vi "SIAM_test_Standalone.vi"() -> ()   [LabVIEW 2011]
uses:
  SIAM_command.ctl
  Library/ScanControl/ScanControl_Action.ctl
  Library/ScanControl/ScanControl_Channel.ctl
  SIAM-send.ctl
  <vilib>/Utility/miscctls.llb/LVRangeTypeDef.ctl
panel:
  in  "Clear":bool
  in  "return":string="78,0,\r\n78,0,\r\n78,0,\r\n78,0,\r\n78,0,\r\n78,0,\r\n78,0,\r\n78,0,\r\n78,0,\r\n78,0,\r\n78,0,\r\n78,0,\r\n78,0,\r\n78,0,\r\n78,0,\r\n78,0,\r\n78,0,\r\n78,0,\r\n78,0,\r\n78,0,\r\n78,0,\r\n78,0,\r\n78,0,\r\n78,0,\r\n78,0,\r\n78,0,\r\n78,0,\r\n78,0,\r\n"
  in  "Registerkarte":T1(tab)
  in  "ScaleConst":T2(array[cluster])=[{"Axis-Ring"=16777217, "Scale"=51200.0, "Offset"=100.0, "HW min"=0.0, "HW max"=5500000.0, "max a"=inf, "units"="mm"}, {"Axis-Ring"=17825793, "Scale"=51200.0, "Offset"=100.0, "HW min"=0.0, "HW max"=3700000.0, "max a"=inf, "units"="mm"}, {"Axis-Ring"=19922945, "Scale"=153600.0, "Offset"=146600.0, "HW min"=0.0, "HW max"=614400.0, "max a"=inf, "units"="Pos"}, {"Axis-Ring"=20971521, "Scale"=25000.1, "Offset"=641.0, "HW min"=0.0, "HW max"=124721.0, "max a"=inf, "units"="Pos"}, {"Axis-Ring"=22020097, "Scale"=1.0, "Offset"=0.0, "HW min"=0.0, "HW max"=51200.0, "max a"=inf, "units"="counts"}, {"Axis-Ring"=23068673, "Scale"=10240.0, "Offset"=0.0, "HW min"=0.0, "HW max"=51200.0, "max a"=inf, "units"="Pos"}, {"Axis-Ring"=24117249, "Scale"=1.0, "Offset"=0.0, "HW min"=0.0, "HW max"=51200.0, "max a"=inf, "units"="counts"}, {"Axis-Ring"=2684354561, "Scale"=1.0, "Offset"=0.0, "HW min"=0.0, "HW max"=65636.0, "max a"=inf, "units"="counts"}, {"Axis-Ring"=2685403137, "Scale"=1.0, "Offset"=0.0, "HW min"=0.0, "HW max"=65636.0, "max a"=inf, "units"="counts"}, {"Axis-Ring"=2686451713, "Scale"=1.0, "Offset"=0.0, "HW min"=0.0, "HW max"=65636.0, "max a"=inf, "units"="counts"}, {"Axis-Ring"=2687500289, "Scale"=1.0, "Offset"=0.0, "HW min"=0.0, "HW max"=65636.0, "max a"=inf, "units"="counts"}, {"Axis-Ring"=2688548865, "Scale"=1.0, "Offset"=0.0, "HW min"=0.0, "HW max"=65636.0, "max a"=inf, "units"="counts"}, {"Axis-Ring"=2689597441, "Scale"=1.0, "Offset"=1.0, "HW min"=0.0, "HW max"=65636.0, "max a"=inf, "units"="counts"}, {"Axis-Ring"=2690646017, "Scale"=1.0, "Offset"=1.0, "HW min"=0.0, "HW max"=65636.0, "max a"=inf, "units"="counts"}, {"Axis-Ring"=2691694593, "Scale"=1.0, "Offset"=1.0, "HW min"=0.0, "HW max"=65636.0, "max a"=inf, "units"="counts"}, {"Axis-Ring"=2701131777, "Scale"=1.0, "Offset"=1.0, "HW min"=0.0, "HW max"=65636.0, "max a"=inf, "units"="counts"}, {"Axis-Ring"=2702180353, "Scale"=1.0, "Offset"=1.0, "HW min"=0.0, "HW max"=65636.0, "max a"=inf, "units"="counts"}, {"Axis-Ring"=2703228929, "Scale"=1.0, "Offset"=1.0, "HW min"=0.0, "HW max"=65636.0, "max a"=inf, "units"="counts"}, {"Axis-Ring"=2704277505, "Scale"=1.0, "Offset"=1.0, "HW min"=0.0, "HW max"=65636.0, "max a"=inf, "units"="counts"}, {"Axis-Ring"=2717908993, "Scale"=1.0, "Offset"=1.0, "HW min"=0.0, "HW max"=65636.0, "max a"=inf, "units"="counts"}, {"Axis-Ring"=2718957569, "Scale"=1.0, "Offset"=1.0, "HW min"=0.0, "HW max"=65636.0, "max a"=inf, "units"="counts"}, {"Axis-Ring"=2720006145, "Scale"=1.0, "Offset"=1.0, "HW min"=0.0, "HW max"=65636.0, "max a"=inf, "units"="counts"}, {"Axis-Ring"=2721054721, "Scale"=1.0, "Offset"=1.0, "HW min"=0.0, "HW max"=65636.0, "max a"=inf, "units"="counts"}, {"Axis-Ring"=67108865, "Scale"=1.0, "Offset"=1.0, "HW min"=100000.0, "HW max"=200000.0, "max a"=inf, "units"="counts"}, {"Axis-Ring"=68157441, "Scale"=1.0, "Offset"=1.0, "HW min"=100000.0, "HW max"=200000.0, "max a"=inf, "units"="counts"}] {"Axis-Ring" items=["X-Axis"=16777217, "Y-Axis"=17825793, "Obj"=19922945, "Filter"=20971521, "Trans"=22020097, "FRET"=23068673, "SI"=24117249, "LED365"=2684354561, "LED385"=2685403137, "LED440"=2686451713, "LED470"=2687500289, "LED510"=2688548865, "LED540"=2689597441, "LED590"=2690646017, "LED640"=2691694593, "DurchR"=2701131777, "DurchG"=2702180353, "DurchB"=2703228929, "AF"=2704277505, "Laser0"=2717908993, "Laser1"=2718957569, "Laser2"=2720006145, "Laser3"=2721054721, "Servo0"=67108865, "Servo1"=68157441]}
  in  "instrument name":string="SAMBoard"
  in  "TMSI-device-scales":T4(array[cluster])=[{"channel"=enum."GalvoX", "m/bit"=8e-07, "min m"=-0.01, "max m"=0.01, "max a [m/s]"=1.0}, {"channel"=enum."GalvoY", "m/bit"=8e-07, "min m"=-0.01, "max m"=0.01, "max a [m/s]"=1.0}, {"channel"=enum."Galvo3", "m/bit"=2e-09, "min m"=-0.01, "max m"=0.02, "max a [m/s]"=1.0}]
  out "Connected":bool
  in  "remote port":u16=3
  in  "address":string="10.153.70.45"
  out "connect error":errorcluster
  in  "Cycletime [s]":dbl=1e-05
  in  "Update length":bool
  out "Elements":i32
  in  "Unroll-loops":bool
  in  "ClearScan":bool
  in  "channel":T3=enum."GalvoX"
  in  "ConvertScan":bool
  in  "Convert String":bool
  in  "Colibri-Scan-String":string="0,0,10,0.00119;0,0,3,-7.2266666667E-5;0,0,4,-8.8133333333E-5;0,0,11,0;0,0,12,0;0,0,7,3;0,4,9,127;0,2,3,0.05875;0,2,4,0;0,2,11,100000;0.00255,2,11,0;0.00256,1,12,1;0.00256,0,7,1;0.00256,2,3,-1.4928955695E-16;0.00256,2,4,0.0073046875;0.00264,0,7,3;0.00264,2,3,-0.05875;0.00264,2,4,0;0.00264,2,11,-100000;0.00519,2,11,0;0.0052,1,12,1;0.0052,0,7,1;0.0052,2,3,1.4928955695E-16;0.0052,2,4,0.0073046875;0.00528,0,7,3;0.00528,5,9,0;0.67056,2,3,0.05875;0.67056,2,4,0;0.67056,2,11,100000;0.67311,2,11,0;0.67312,1,12,1;0.67312,0,7,1;0.67312,2,3,-1.4928955695E-16;0.67312,2,4,0.0073046875;0.6732,0,7,3;0.6732,2,3,-0.05875;0.6732,2,4,0;0.6732,2,11,-100000;0.67575,2,11,0;0.67576,2,3,0;0.67576,2,4,0;0.67576,0,7,0;"
  in  "ScanSteuerung":T6(array[cluster])
  in  "Frequency [Hz]":dbl=500.0
  in  "duration [s]":dbl=1.0
  in  "Amplitude \n(count pk-pk)":dbl=6553.6 format="%#_5g"
  in  "Create":bool
  in  "Offset [count]":dbl=1.0
  in  "Range":bool
  in  "+-Range":i32=1000
  in  "Position":i32(slide) scale=-32000.0..32000.0
  in  "Motor":T7(ring)
  in  "Axis":T8={"Linear"={"Axis-Ring"=16777217, "Position"=0}, "Linear"={"Axis-Ring"=17825793, "Position"=0}, "Linear 2"={"Axis-Ring"=19922945, "Position"=0}, "Linear 3"={"Axis-Ring"=20971521, "Position"=0}, "Linear"={"Axis-Ring"=22020097, "Position"=0}, "Linear 4"={"Axis-Ring"=2684354561, "Position"=0}, "Linear 5"={"Axis-Ring"=2685403137, "Position"=0}, "Linear 6"={"Axis-Ring"=2687500289, "Position"=0}, "Linear 7"={"Axis-Ring"=2691694593, "Position"=0}, "Linear 8"={"Axis-Ring"=2701131777, "Position"=0}, "Linear 9"={"Axis-Ring"=2717908993, "Position"=0}, "Linear 10"={"Axis-Ring"=2718957569, "Position"=0}, "Linear 11"={"Axis-Ring"=2720006145, "Position"=0}, "Linear 12"={"Axis-Ring"=2721054721, "Position"=0}, "Linear 13"={"Axis-Ring"=67108865, "Position"=150000}} {"Linear 13"."Axis-Ring" items=["X-Axis"=16777217, "Y-Axis"=17825793, "Obj"=19922945, "Filter"=20971521, "Trans"=22020097, "FRET"=23068673, "SI"=24117249, "LED365"=2684354561, "LED385"=2685403137, "LED440"=2686451713, "LED470"=2687500289, "LED510"=2688548865, "LED540"=2689597441, "LED590"=2690646017, "LED640"=2691694593, "DurchR"=2701131777, "DurchG"=2702180353, "DurchB"=2703228929, "AF"=2704277505, "Laser0"=2717908993, "Laser1"=2718957569, "Laser2"=2720006145, "Laser3"=2721054721, "Servo0"=67108865, "Servo1"=68157441]; "Linear 13"."Position" scale=100000.0..200000.0; "Linear 12"."Axis-Ring" items=["X-Axis"=16777217, "Y-Axis"=17825793, "Obj"=19922945, "Filter"=20971521, "Trans"=22020097, "FRET"=23068673, "SI"=24117249, "LED365"=2684354561, "LED385"=2685403137, "LED440"=2686451713, "LED470"=2687500289, "LED510"=2688548865, "LED540"=2689597441, "LED590"=2690646017, "LED640"=2691694593, "DurchR"=2701131777, "DurchG"=2702180353, "DurchB"=2703228929, "AF"=2704277505, "Laser0"=2717908993, "Laser1"=2718957569, "Laser2"=2720006145, "Laser3"=2721054721, "Servo0"=67108865, "Servo1"=68157441]; "Linear 12"."Position" scale=0.0..65000.0; "Linear 11"."Axis-Ring" items=["X-Axis"=16777217, "Y-Axis"=17825793, "Obj"=19922945, "Filter"=20971521, "Trans"=22020097, "FRET"=23068673, "SI"=24117249, "LED365"=2684354561, "LED385"=2685403137, "LED440"=2686451713, "LED470"=2687500289, "LED510"=2688548865, "LED540"=2689597441, "LED590"=2690646017, "LED640"=2691694593, "DurchR"=2701131777, "DurchG"=2702180353, "DurchB"=2703228929, "AF"=2704277505, "Laser0"=2717908993, "Laser1"=2718957569, "Laser2"=2720006145, "Laser3"=2721054721, "Servo0"=67108865, "Servo1"=68157441]; "Linear 11"."Position" scale=0.0..65000.0; "Linear 10"."Axis-Ring" items=["X-Axis"=16777217, "Y-Axis"=17825793, "Obj"=19922945, "Filter"=20971521, "Trans"=22020097, "FRET"=23068673, "SI"=24117249, "LED365"=2684354561, "LED385"=2685403137, "LED440"=2686451713, "LED470"=2687500289, "LED510"=2688548865, "LED540"=2689597441, "LED590"=2690646017, "LED640"=2691694593, "DurchR"=2701131777, "DurchG"=2702180353, "DurchB"=2703228929, "AF"=2704277505, "Laser0"=2717908993, "Laser1"=2718957569, "Laser2"=2720006145, "Laser3"=2721054721, "Servo0"=67108865, "Servo1"=68157441]; "Linear 10"."Position" scale=0.0..65000.0; "Linear 9"."Axis-Ring" items=["X-Axis"=16777217, "Y-Axis"=17825793, "Obj"=19922945, "Filter"=20971521, "Trans"=22020097, "FRET"=23068673, "SI"=24117249, "LED365"=2684354561, "LED385"=2685403137, "LED440"=2686451713, "LED470"=2687500289, "LED510"=2688548865, "LED540"=2689597441, "LED590"=2690646017, "LED640"=2691694593, "DurchR"=2701131777, "DurchG"=2702180353, "DurchB"=2703228929, "AF"=2704277505, "Laser0"=2717908993, "Laser1"=2718957569, "Laser2"=2720006145, "Laser3"=2721054721, "Servo0"=67108865, "Servo1"=68157441]; "Linear 9"."Position" scale=0.0..65000.0; "Linear 8"."Axis-Ring" items=["X-Axis"=16777217, "Y-Axis"=17825793, "Obj"=19922945, "Filter"=20971521, "Trans"=22020097, "FRET"=23068673, "SI"=24117249, "LED365"=2684354561, "LED385"=2685403137, "LED440"=2686451713, "LED470"=2687500289, "LED510"=2688548865, "LED540"=2689597441, "LED590"=2690646017, "LED640"=2691694593, "DurchR"=2701131777, "DurchG"=2702180353, "DurchB"=2703228929, "AF"=2704277505, "Laser0"=2717908993, "Laser1"=2718957569, "Laser2"=2720006145, "Laser3"=2721054721, "Servo0"=67108865, "Servo1"=68157441]; "Linear 8"."Position" scale=0.0..65000.0; "Linear 7"."Axis-Ring" items=["X-Axis"=16777217, "Y-Axis"=17825793, "Obj"=19922945, "Filter"=20971521, "Trans"=22020097, "FRET"=23068673, "SI"=24117249, "LED365"=2684354561, "LED385"=2685403137, "LED440"=2686451713, "LED470"=2687500289, "LED510"=2688548865, "LED540"=2689597441, "LED590"=2690646017, "LED640"=2691694593, "DurchR"=2701131777, "DurchG"=2702180353, "DurchB"=2703228929, "AF"=2704277505, "Laser0"=2717908993, "Laser1"=2718957569, "Laser2"=2720006145, "Laser3"=2721054721, "Servo0"=67108865, "Servo1"=68157441]; "Linear 7"."Position" scale=0.0..65000.0; "Linear 6"."Axis-Ring" items=["X-Axis"=16777217, "Y-Axis"=17825793, "Obj"=19922945, "Filter"=20971521, "Trans"=22020097, "FRET"=23068673, "SI"=24117249, "LED365"=2684354561, "LED385"=2685403137, "LED440"=2686451713, "LED470"=2687500289, "LED510"=2688548865, "LED540"=2689597441, "LED590"=2690646017, "LED640"=2691694593, "DurchR"=2701131777, "DurchG"=2702180353, "DurchB"=2703228929, "AF"=2704277505, "Laser0"=2717908993, "Laser1"=2718957569, "Laser2"=2720006145, "Laser3"=2721054721, "Servo0"=67108865, "Servo1"=68157441]; "Linear 6"."Position" scale=0.0..65000.0; "Linear 5"."Axis-Ring" items=["X-Axis"=16777217, "Y-Axis"=17825793, "Obj"=19922945, "Filter"=20971521, "Trans"=22020097, "FRET"=23068673, "SI"=24117249, "LED365"=2684354561, "LED385"=2685403137, "LED440"=2686451713, "LED470"=2687500289, "LED510"=2688548865, "LED540"=2689597441, "LED590"=2690646017, "LED640"=2691694593, "DurchR"=2701131777, "DurchG"=2702180353, "DurchB"=2703228929, "AF"=2704277505, "Laser0"=2717908993, "Laser1"=2718957569, "Laser2"=2720006145, "Laser3"=2721054721, "Servo0"=67108865, "Servo1"=68157441]; "Linear 5"."Position" scale=0.0..65000.0; "Linear 4"."Axis-Ring" items=["X-Axis"=16777217, "Y-Axis"=17825793, "Obj"=19922945, "Filter"=20971521, "Trans"=22020097, "FRET"=23068673, "SI"=24117249, "LED365"=2684354561, "LED385"=2685403137, "LED440"=2686451713, "LED470"=2687500289, "LED510"=2688548865, "LED540"=2689597441, "LED590"=2690646017, "LED640"=2691694593, "DurchR"=2701131777, "DurchG"=2702180353, "DurchB"=2703228929, "AF"=2704277505, "Laser0"=2717908993, "Laser1"=2718957569, "Laser2"=2720006145, "Laser3"=2721054721, "Servo0"=67108865, "Servo1"=68157441]; "Linear 4"."Position" scale=0.0..65000.0; "Linear"."Axis-Ring" items=["X-Axis"=16777217, "Y-Axis"=17825793, "Obj"=19922945, "Filter"=20971521, "Trans"=22020097, "FRET"=23068673, "SI"=24117249, "LED365"=2684354561, "LED385"=2685403137, "LED440"=2686451713, "LED470"=2687500289, "LED510"=2688548865, "LED540"=2689597441, "LED590"=2690646017, "LED640"=2691694593, "DurchR"=2701131777, "DurchG"=2702180353, "DurchB"=2703228929, "AF"=2704277505, "Laser0"=2717908993, "Laser1"=2718957569, "Laser2"=2720006145, "Laser3"=2721054721, "Servo0"=67108865, "Servo1"=68157441]; "Linear"."Position" scale=0.0..51200.0; "Linear 3"."Axis-Ring" items=["X-Axis"=16777217, "Y-Axis"=17825793, "Obj"=19922945, "Filter"=20971521, "Trans"=22020097, "FRET"=23068673, "SI"=24117249, "LED365"=2684354561, "LED385"=2685403137, "LED440"=2686451713, "LED470"=2687500289, "LED510"=2688548865, "LED540"=2689597441, "LED590"=2690646017, "LED640"=2691694593, "DurchR"=2701131777, "DurchG"=2702180353, "DurchB"=2703228929, "AF"=2704277505, "Laser0"=2717908993, "Laser1"=2718957569, "Laser2"=2720006145, "Laser3"=2721054721, "Servo0"=67108865, "Servo1"=68157441]; "Linear 3"."Position" scale=0.0..124700.0; "Linear 2"."Axis-Ring" items=["X-Axis"=16777217, "Y-Axis"=17825793, "Obj"=19922945, "Filter"=20971521, "Trans"=22020097, "FRET"=23068673, "SI"=24117249, "LED365"=2684354561, "LED385"=2685403137, "LED440"=2686451713, "LED470"=2687500289, "LED510"=2688548865, "LED540"=2689597441, "LED590"=2690646017, "LED640"=2691694593, "DurchR"=2701131777, "DurchG"=2702180353, "DurchB"=2703228929, "AF"=2704277505, "Laser0"=2717908993, "Laser1"=2718957569, "Laser2"=2720006145, "Laser3"=2721054721, "Servo0"=67108865, "Servo1"=68157441]; "Linear 2"."Position" scale=0.0..614400.0; "Linear"."Axis-Ring" items=["X-Axis"=16777217, "Y-Axis"=17825793, "Obj"=19922945, "Filter"=20971521, "Trans"=22020097, "FRET"=23068673, "SI"=24117249, "LED365"=2684354561, "LED385"=2685403137, "LED440"=2686451713, "LED470"=2687500289, "LED510"=2688548865, "LED540"=2689597441, "LED590"=2690646017, "LED640"=2691694593, "DurchR"=2701131777, "DurchG"=2702180353, "DurchB"=2703228929, "AF"=2704277505, "Laser0"=2717908993, "Laser1"=2718957569, "Laser2"=2720006145, "Laser3"=2721054721, "Servo0"=67108865, "Servo1"=68157441]; "Linear"."Position" scale=0.0..3500000.0; "Linear"."Axis-Ring" items=["X-Axis"=16777217, "Y-Axis"=17825793, "Obj"=19922945, "Filter"=20971521, "Trans"=22020097, "FRET"=23068673, "SI"=24117249, "LED365"=2684354561, "LED385"=2685403137, "LED440"=2686451713, "LED470"=2687500289, "LED510"=2688548865, "LED540"=2689597441, "LED590"=2690646017, "LED640"=2691694593, "DurchR"=2701131777, "DurchG"=2702180353, "DurchB"=2703228929, "AF"=2704277505, "Laser0"=2717908993, "Laser1"=2718957569, "Laser2"=2720006145, "Laser3"=2721054721, "Servo0"=67108865, "Servo1"=68157441]; "Linear"."Position" scale=0.0..5500000.0}
  in  "Array":T9(array[cluster])=[{"Digital-out"=enum."cam1", "Boolean"=FALSE}, {"Digital-out"=enum."led1", "Boolean"=FALSE}, {"Digital-out"=enum."led2", "Boolean"=FALSE}, {"Digital-out"=enum."led3", "Boolean"=FALSE}, {"Digital-out"=enum."led4", "Boolean"=FALSE}, {"Digital-out"=enum."led5", "Boolean"=FALSE}, {"Digital-out"=enum."led5", "Boolean"=FALSE}, {"Digital-out"=enum."led7", "Boolean"=FALSE}, {"Digital-out"=enum."led8", "Boolean"=FALSE}, {"Digital-out"=enum."durchR", "Boolean"=FALSE}, {"Digital-out"=enum."durchG", "Boolean"=FALSE}, {"Digital-out"=enum."durchB", "Boolean"=FALSE}, {"Digital-out"=enum."AF", "Boolean"=FALSE}, {"Digital-out"=enum."Laser0", "Boolean"=FALSE}, {"Digital-out"=enum."Laser1", "Boolean"=FALSE}, {"Digital-out"=enum."Laser2", "Boolean"=FALSE}, {"Digital-out"=enum."Laser3", "Boolean"=FALSE}, {"Digital-out"=enum."TrigOut", "Boolean"=FALSE}, {"Digital-out"=enum."SMB1", "Boolean"=FALSE}]
  in  "Run":bool
  in  "SendScript":bool
  in  "Load":bool
  in  "Save":bool
  in  "ClearScript":bool
  in  "Script":T11(array[cluster])=[{"Delay 10µs"=0, "command"=4027514895, "P0"=0, "P1"=0, "P2"=0, "P3"=0, "P4"=0, "P5-ticket"=0}] {"command" format="%x" items=["read_x-Motor_status_ticket"=17305600, "init_x-Motor"=17760263, "read_x-Motor_absolute_ticket"=16781312, "move_x-Motor_absolute"=16777217, "move_x-Motor_relative"=16842753, "read_x-Motor_speed"=16977920, "set_x-Motor_speed"=16973825, "read_y-Motor_status_ticket"=18354176, "init_y-Motor"=18808839, "read_y-Motor_absolute_ticket"=17829888, "move_y-Motor_absolute"=17825793, "move_y-Motor_relative"=17891329, "read_y-Motor_speed"=18026496, "set_y-Motor_speed"=18022401, "read_z-Motor_status_ticket"=19402752, "init_z-Motor"=19857415, "stop_z-Motor"=19857423, "start_z-Motor"=19857422, "read_z-Motor_absolute_ticket"=18878464, "move_z-Motor_absolute"=18874369, "move_z-Motor_relative"=18939905, "read_Objective_status_ticket"=20451328, "init_Objective"=20905991, "read_Objective_absolute_ticket"=19927040, "move_Objective_absolute"=19922945, "move_Objective_relative"=19988481, "read_Objective-Motor_speed"=20123648, "set_Objective-Motor_speed"=20119553, "read_Filter_status_ticket"=21499904, "init_Filter"=21954567, "read_Filter_absolute_ticket"=20975616, "move_Filter_absolute"=20971521, "move_Filter_relative"=21037057, "read_Filter-Motor_speed"=21172224, "set_Filter-Motor_speed"=21168129, "read_Trans-Rad_status_ticket"=22548480, "init_Trans-Rad"=23003143, "read_Trans-Rad_absolute_ticket"=22024192, "move_Trans-Rad_absolute"=22020097, "move_Trans-Rad_relative"=22085633, "read_Trans-Motor_speed"=22220800, "set_Trans-Motor_speed"=22216705, "read_FRET_status_ticket"=23597056, "init_FRET"=24051719, "read_FRET_absolute_ticket"=23072768, "move_FRET_absolute"=23068673, "move_FRET_relative"=23134209, "read_FRET-Motor_speed"=23269376, "set_FRET-Motor_speed"=23265281, "read_SI-Rad_status_ticket"=24645632, "init_SI-Rad"=25100295, "read_SI-Rad_absolute_ticket"=24121344, "move_SI-Rad_absolute"=24117249, "move_SI-Rad_relative"=24182785, "read_SI-Rad_speed"=24317952, "set_SI-Rad_speed"=24313857, "end_no_ticket"=4027514895, "end_ticket"=4027518991, "IO-read_bank0"=3489665024, "IO-write_bank0"=3489660929, "IO-read_bank1"=3506442240, "IO-write_bank1"=3506438145, "DA0-0_LED365"=2684354561, "DA0-1_LED385"=2685403137, "DA0-2_LED440"=2686451713, "DA0-3_LED470"=2687500289, "DA0-4_LED510"=2688548865, "DA0-5_LED550"=2689597441, "DA0-6_LED590"=2690646017, "DA0-7_LED640"=2691694593, "DA1-0_LED-R"=2701131777, "DA1-1_LED-G"=2702180353, "DA1-2_LED-B"=2703228929, "DA1-3_LED-AF"=2704277505, "DA1-4"=2705326081, "DA1-5"=2706374657, "DA1-6"=2707423233, "DA1-7"=2708471809, "DA2-Laser0"=2717908993, "DA2-Laser1"=2718957569, "DA2-Laser2"=2720006145, "DA2-Laser3"=2721054721, "DA2-Laser4"=2722103297, "Analog-read_AD0-0"=2818576384, "Analog-read-store_AD0-0"=2818572290, "IO-delay_bank0"=3489923073, "IO-delay_bank0_fromVar"=3489923075, "read_cam_clock"=3289124864, "store_cam_clock"=3289120770, "read_cam_phase"=3289190400, "store_cam_phase"=3289190402, "Read ticks"=4027518976, "Read ticks to var"=4027518978, "Read IP"=4043313152, "Read IP into var"=4043313154, "Set IP from var"=4043309059, "Set IP from var, relative"=4043313155, "decrement_branchRel_if_equal"=4043374945, "decrement_branchRel_if_greaterequal"=4043375201, "decrement_branchRel_if_greaterequal_withTicket"=4043379297, "decrement_branchRel_if_smaller"=4043375457, "increment_branchRel_if_smaller"=4043375473, "readVar"=4060090368, "writeVar"=4060086273, "readVar_and_copy_to_var2"=4060086275, "loadVar2_andcopy_var1"=4060086276, "math_addToVariable"=4076863488, "math_addVToVariable"=4076863489, "math_subToVariable"=4076863490, "math_subVToVariable"=4076863491, "math_multToVariable"=4076863492, "math_multvToVariable"=4076863493, "math_divideToVariable"=4076863494, "math_divideVToVariable"=4076863495, "math_modToVariable"=4076863496, "math_modVToVariable"=4076863497, "logic_and"=4093640704, "logic_or"=4093640706, "logic_xor"=4093640708, "set_1Galvo"=101712113, "set_x-Galvo"=102760689, "set_y-Galvo"=103809265, "set_z-Fokus"=104857841, "set_1Galvo_position-only"=101711937, "set_x-Galvo_position-only"=102760513, "set_y-Galvo_position-only"=103809089, "set_z-Fokus_position-only"=104857665, "set_x-Galvo_position-only_ticket"=102764609, "set_y-Galvo_position-only_ticket"=103813185, "set_z-Fokus_position-only_ticket"=104861761, "set_x-Galvo_relativ-only"=102760577, "set_y-Galvo_relativ-only"=103809153, "set_z-Fokus_relativ-only"=104857729, "set_x-Galvo_speed-only"=102760481, "set_y-Galvo_speed-only"=103809057, "set_z-Fokus_speed-only"=104857633, "read_1Galvo_ticket"=101716032, "read_x-Galvo_ticket"=102764608, "read_y-Galvo_ticket"=103813184, "read_z-Focus_ticket"=104861760, "x-Galvo_pos_fromVar"=102760515, "y-Galvo_pos_fromVar"=103809091, "z-Focus_pos_fromVar"=104857667, "Servo0"=67108865, "Servo0-enable"=68091911, "Servo0-disable"=68091919, "Servo1"=68157441, "Servo1-enable"=69140487, "Servo1-disable"=69140495, "EnablePower0-SM"=2148466695, "DisablePower0-SM"=2148466703, "EnablePower1-Thermo1"=2149515271, "DisablePower1-Thermo1"=2149515279, "EnablePower2-Cam"=2150563847, "DisablePower2-Cam"=2150563855, "EnablePower3-Thermo2"=2151612423, "DisablePower3-Thermo2"=2151612431, "EnablePower4-Laser0"=2152660999, "DisablePower4-Laser0"=2152661007, "EnablePower5"=2153709575, "DisablePower5"=2153709583, "EnablePower6-Laser1"=2154758151, "DisablePower6-Laser1"=2154758159, "EnablePower7-SAM"=2155806727, "DisablePower7-SAM"=2155806735, "EnablePower8-Laser2"=2156855303, "DisablePower8-Laser2"=2156855311, "EnablePower9-TSM"=2157903879, "DisablePower9-TSM"=2157903887, "EnablePower10-Laser3"=2158952455, "DisablePower10-Laser3"=2158952463, "EnablePower11-Servo"=2160001031, "DisablePower11-Servo"=2160001039, "EnablePower12-Laser4"=2161049607, "DisablePower12-Laser4"=2161049615, "EnableSMPower2-DCC22"=2167341063, "DisableSMPower2-DCC22"=2167341071, "EnableSMPower3-6220"=2168389639, "DisableSMPower3-6220"=2168389647, "EnableSMPower4-6210"=2169438215, "DisableSMPower4-6210"=2169438223]; "P5-ticket" format="%.0x"; "Delay 10µs" format="%.0x"; "P1" format="%.0x"}
  in  "Cluster":T12={"Delay 10µs"=0, "command"=17760263, "P0"=1, "P1"=0, "P2"=0, "P3"=0, "P4"=0, "P5-ticket"=0} {"command" format="%x" items=["read_x-Motor_status_ticket"=17305600, "init_x-Motor"=17760263, "read_x-Motor_absolute_ticket"=16781312, "move_x-Motor_absolute"=16777217, "move_x-Motor_relative"=16842753, "read_x-Motor_speed"=16977920, "set_x-Motor_speed"=16973825, "read_y-Motor_status_ticket"=18354176, "init_y-Motor"=18808839, "read_y-Motor_absolute_ticket"=17829888, "move_y-Motor_absolute"=17825793, "move_y-Motor_relative"=17891329, "read_y-Motor_speed"=18026496, "set_y-Motor_speed"=18022401, "read_z-Motor_status_ticket"=19402752, "init_z-Motor"=19857415, "stop_z-Motor"=19857423, "start_z-Motor"=19857422, "read_z-Motor_absolute_ticket"=18878464, "move_z-Motor_absolute"=18874369, "move_z-Motor_relative"=18939905, "read_Objective_status_ticket"=20451328, "init_Objective"=20905991, "read_Objective_absolute_ticket"=19927040, "move_Objective_absolute"=19922945, "move_Objective_relative"=19988481, "read_Objective-Motor_speed"=20123648, "set_Objective-Motor_speed"=20119553, "read_Filter_status_ticket"=21499904, "init_Filter"=21954567, "read_Filter_absolute_ticket"=20975616, "move_Filter_absolute"=20971521, "move_Filter_relative"=21037057, "read_Filter-Motor_speed"=21172224, "set_Filter-Motor_speed"=21168129, "read_Trans-Rad_status_ticket"=22548480, "init_Trans-Rad"=23003143, "read_Trans-Rad_absolute_ticket"=22024192, "move_Trans-Rad_absolute"=22020097, "move_Trans-Rad_relative"=22085633, "read_Trans-Motor_speed"=22220800, "set_Trans-Motor_speed"=22216705, "read_FRET_status_ticket"=23597056, "init_FRET"=24051719, "read_FRET_absolute_ticket"=23072768, "move_FRET_absolute"=23068673, "move_FRET_relative"=23134209, "read_FRET-Motor_speed"=23269376, "set_FRET-Motor_speed"=23265281, "read_SI-Rad_status_ticket"=24645632, "init_SI-Rad"=25100295, "read_SI-Rad_absolute_ticket"=24121344, "move_SI-Rad_absolute"=24117249, "move_SI-Rad_relative"=24182785, "read_SI-Rad_speed"=24317952, "set_SI-Rad_speed"=24313857, "end_no_ticket"=4027514895, "end_ticket"=4027518991, "IO-read_bank0"=3489665024, "IO-write_bank0"=3489660929, "IO-read_bank1"=3506442240, "IO-write_bank1"=3506438145, "DA0-0_LED365"=2684354561, "DA0-1_LED385"=2685403137, "DA0-2_LED440"=2686451713, "DA0-3_LED470"=2687500289, "DA0-4_LED510"=2688548865, "DA0-5_LED550"=2689597441, "DA0-6_LED590"=2690646017, "DA0-7_LED640"=2691694593, "DA1-0_LED-R"=2701131777, "DA1-1_LED-G"=2702180353, "DA1-2_LED-B"=2703228929, "DA1-3_LED-AF"=2704277505, "DA1-4"=2705326081, "DA1-5"=2706374657, "DA1-6"=2707423233, "DA1-7"=2708471809, "DA2-Laser0"=2717908993, "DA2-Laser1"=2718957569, "DA2-Laser2"=2720006145, "DA2-Laser3"=2721054721, "DA2-Laser4"=2722103297, "Analog-read_AD0-0"=2818576384, "Analog-read-store_AD0-0"=2818572290, "IO-delay_bank0"=3489923073, "IO-delay_bank0_fromVar"=3489923075, "read_cam_clock"=3289124864, "store_cam_clock"=3289120770, "read_cam_phase"=3289190400, "store_cam_phase"=3289190402, "Read ticks"=4027518976, "Read ticks to var"=4027518978, "Read IP"=4043313152, "Read IP into var"=4043313154, "Set IP from var"=4043309059, "Set IP from var, relative"=4043313155, "decrement_branchRel_if_equal"=4043374945, "decrement_branchRel_if_greaterequal"=4043375201, "decrement_branchRel_if_greaterequal_withTicket"=4043379297, "decrement_branchRel_if_smaller"=4043375457, "increment_branchRel_if_smaller"=4043375473, "readVar"=4060090368, "writeVar"=4060086273, "readVar_and_copy_to_var2"=4060086275, "loadVar2_andcopy_var1"=4060086276, "math_addToVariable"=4076863488, "math_addVToVariable"=4076863489, "math_subToVariable"=4076863490, "math_subVToVariable"=4076863491, "math_multToVariable"=4076863492, "math_multvToVariable"=4076863493, "math_divideToVariable"=4076863494, "math_divideVToVariable"=4076863495, "math_modToVariable"=4076863496, "math_modVToVariable"=4076863497, "logic_and"=4093640704, "logic_or"=4093640706, "logic_xor"=4093640708, "set_1Galvo"=101712113, "set_x-Galvo"=102760689, "set_y-Galvo"=103809265, "set_z-Fokus"=104857841, "set_1Galvo_position-only"=101711937, "set_x-Galvo_position-only"=102760513, "set_y-Galvo_position-only"=103809089, "set_z-Fokus_position-only"=104857665, "set_x-Galvo_position-only_ticket"=102764609, "set_y-Galvo_position-only_ticket"=103813185, "set_z-Fokus_position-only_ticket"=104861761, "set_x-Galvo_relativ-only"=102760577, "set_y-Galvo_relativ-only"=103809153, "set_z-Fokus_relativ-only"=104857729, "set_x-Galvo_speed-only"=102760481, "set_y-Galvo_speed-only"=103809057, "set_z-Fokus_speed-only"=104857633, "read_1Galvo_ticket"=101716032, "read_x-Galvo_ticket"=102764608, "read_y-Galvo_ticket"=103813184, "read_z-Focus_ticket"=104861760, "x-Galvo_pos_fromVar"=102760515, "y-Galvo_pos_fromVar"=103809091, "z-Focus_pos_fromVar"=104857667, "Servo0"=67108865, "Servo0-enable"=68091911, "Servo0-disable"=68091919, "Servo1"=68157441, "Servo1-enable"=69140487, "Servo1-disable"=69140495, "EnablePower0-SM"=2148466695, "DisablePower0-SM"=2148466703, "EnablePower1-Thermo1"=2149515271, "DisablePower1-Thermo1"=2149515279, "EnablePower2-Cam"=2150563847, "DisablePower2-Cam"=2150563855, "EnablePower3-Thermo2"=2151612423, "DisablePower3-Thermo2"=2151612431, "EnablePower4-Laser0"=2152660999, "DisablePower4-Laser0"=2152661007, "EnablePower5"=2153709575, "DisablePower5"=2153709583, "EnablePower6-Laser1"=2154758151, "DisablePower6-Laser1"=2154758159, "EnablePower7-SAM"=2155806727, "DisablePower7-SAM"=2155806735, "EnablePower8-Laser2"=2156855303, "DisablePower8-Laser2"=2156855311, "EnablePower9-TSM"=2157903879, "DisablePower9-TSM"=2157903887, "EnablePower10-Laser3"=2158952455, "DisablePower10-Laser3"=2158952463, "EnablePower11-Servo"=2160001031, "DisablePower11-Servo"=2160001039, "EnablePower12-Laser4"=2161049607, "DisablePower12-Laser4"=2161049615, "EnableSMPower2-DCC22"=2167341063, "DisableSMPower2-DCC22"=2167341071, "EnableSMPower3-6220"=2168389639, "DisableSMPower3-6220"=2168389647, "EnableSMPower4-6210"=2169438215, "DisableSMPower4-6210"=2169438223]; "P5-ticket" format="%.0x"; "Delay 10µs" format="%.0x"; "P0" format="%.0x"; "P1" format="%.0x"}
  in  "WrapperCommands":u16(ring)=100 format="%x" items=["Stop"=112, "ReInit FPGA"=49, "Clear Error"=67, "Dump registers"=100, "Dump memory"=68]
  in  "Wrapper":bool
  in  "Special":bool
  in  "Value":i32
  in  "special send options":T13=enum."rundirect"
  out "Return":i32[](array[numeric])=[120, 0] format="%.0x"
  out "send error":errorcluster
  out "recieve error":errorcluster={"status"=TRUE, "code"=66, "source"="TCP Read in SIAM_test_Standalone2.vi"}
  in  "MotorScale":cluster{"Scale.Range":T14, "Value":i32}[](array[cluster])=[{"Scale.Range"={"Minimum"=-32000.0, "Maximum"=32000.0, "Increment"=20000.0, "Minor Increment"=2000.0, "Start"=-20000.0}, "Value"=0}, {"Scale.Range"={"Minimum"=-32000.0, "Maximum"=32000.0, "Increment"=50000.0, "Minor Increment"=5000.0, "Start"=0.0}, "Value"=0}, {"Scale.Range"={"Minimum"=-12500.0, "Maximum"=0.0, "Increment"=2500.0, "Minor Increment"=500.0, "Start"=-12500.0}, "Value"=0}, {"Scale.Range"={"Minimum"=-32000.0, "Maximum"=32000.0, "Increment"=50000.0, "Minor Increment"=5000.0, "Start"=0.0}, "Value"=0}, {"Scale.Range"={"Minimum"=-4967000.0, "Maximum"=-4750000.0, "Increment"=50000.0, "Minor Increment"=10000.0, "Start"=-4950000.0}, "Value"=-4865332}]
  in  "End":bool
  # "enter before execution"
  # "better this constants, for each device?\nGalvo +-30°opt,f=50mm: 7.9897E-7 m/count"
  # "HW=val*scale+offset"
  # "scale    offset   min max maxa  name"
  # "Triangle-Ramps"
  # "TMSI-Direkt:"
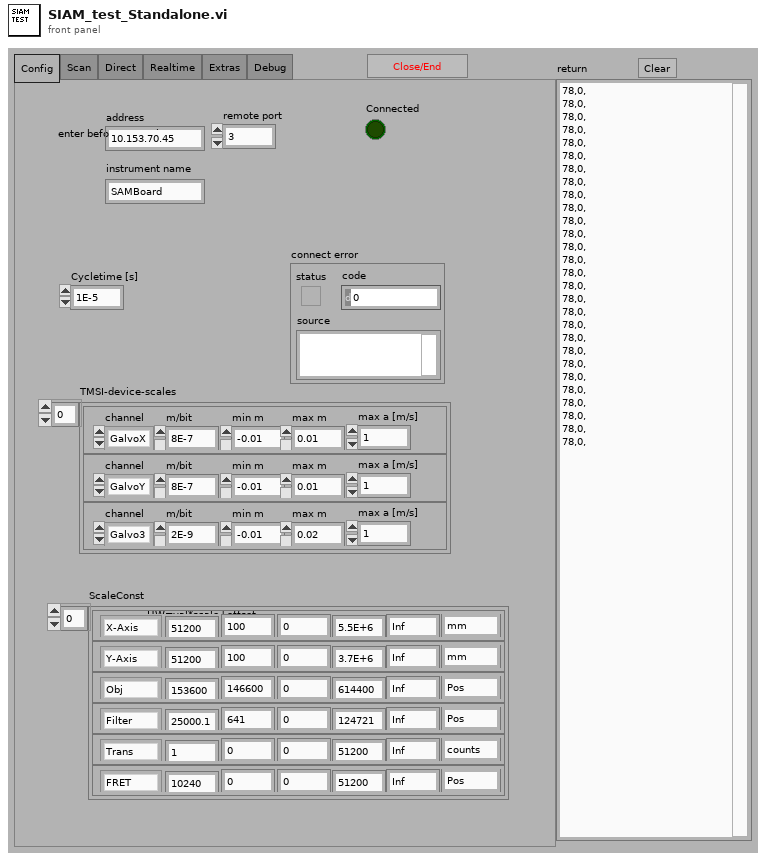
[diagram p1: front panel]
types:
  T1 = enum32{"Config", "Scan", "Direct", "Realtime", "Extras", "Debug"}
  T2 = cluster{"Axis-Ring":u32, "Scale":dbl, "Offset":dbl, "HW min":dbl, "HW max":dbl, "max a":dbl, "units":string}[]
  T3 = typedef "ScanControl_Channel.ctl" = enum16{"Com", "AnalogConfig", "AnalogValue", "GalvoX", "GalvoY", "Galvo3", "Galvo4", "Digital", "Free", "Loop", "SMoveTime", "Image1X", "Image1Y", "Image2X", "Image2Y"}
  T4 = cluster{"channel":T3, "m/bit":dbl, "min m":dbl, "max m":dbl, "max a [m/s]":dbl}[]
  T5 = typedef "ScanControl_Action.ctl" = enum16{"Abs", "Rel", "Inc", "IncInc", "LoopStart", "LoopEnd", "WaitTriggerRising"}
  T6 = cluster{"Time [s]":dbl, "action":T5, "channel":T3, "value (m/s)":dbl}[]
  T7 = enum16{"Ch0", "Ch1", "x-Galvo", "y-Galvo", "z-Focus"}
  T8 = cluster{"Linear":cluster{"Axis-Ring":u32, "Position":i32}, "Linear":cluster{"Axis-Ring":u32, "Position":i32}, "Linear 2":cluster{"Axis-Ring":u32, "Position":i32}, "Linear 3":cluster{"Axis-Ring":u32, "Position":i32}, "Linear":cluster{"Axis-Ring":u32, "Position":i32}, "Linear 4":cluster{"Axis-Ring":u32, "Position":i32}, "Linear 5":cluster{"Axis-Ring":u32, "Position":i32}, "Linear 6":cluster{"Axis-Ring":u32, "Position":i32}, "Linear 7":cluster{"Axis-Ring":u32, "Position":i32}, "Linear 8":cluster{"Axis-Ring":u32, "Position":i32}, "Linear 9":cluster{"Axis-Ring":u32, "Position":i32}, "Linear 10":cluster{"Axis-Ring":u32, "Position":i32}, "Linear 11":cluster{"Axis-Ring":u32, "Position":i32}, "Linear 12":cluster{"Axis-Ring":u32, "Position":i32}, "Linear 13":cluster{"Axis-Ring":u32, "Position":i32}}
  T9 = cluster{"Digital-out":enum8{"cam1", "cam1-ready?", "cam2", "cam2-ready?", "tmsx?", "tsmy?", "tsm3?", "lid?", "led1", "led2", "led3", "led4", "led5", "led6", "led7", "led8", "durchR", "durchG", "durchB", "AF", "Laser0", "Laser1", "Laser2", "Laser3", "Laser4", "LaserX", "TrigOut", "SMB1", ""}, "Boolean":bool}[]
  T10 = typedef "SIAM_command.ctl" = u32
  T11 = cluster{"Delay 10µs":u32, "command":T10, "P0":i32, "P1":i32, "P2":i32, "P3":i32, "P4":i32, "P5-ticket":i32}[]
  T12 = cluster{"Delay 10µs":u32, "command":T10, "P0":i32, "P1":i32, "P2":i32, "P3":i32, "P4":i32, "P5-ticket":i32}
  T13 = typedef "SIAM-send.ctl" = enum16{"validID", "storeID", "enable", "rundirect", "sendlist", "run", "stop", "readRegister", "sendValue", "storeStatus"}
  T14 = typedef "LVRangeTypeDef.ctl" = cluster{"Minimum":dbl, "Maximum":dbl, "Increment":dbl, "Minor Increment":dbl, "Start":dbl}
  T15 = enum16{"Standard", "Buffered", "CRLF", "Immediate"}
  T16 = cluster{"rel 10µs":u32, "Device":T10, "data0":i32, "data1":i32, "data2":i32, "data3":i32, "data4":i32, "data5":i32}
  T17 = enum16{"triangle", "fixed xy-circle", "fixed xy-square"}
  T18 = cluster{"Time [s]":dbl, "action":T5, "channel":T3, "value (/s)":dbl}[]
  T19 = enum8{"cam1", "cam1-ready?", "cam2", "cam2-ready?", "tmsx?", "tsmy?", "tsm3?", "lid?", "led1", "led2", "led3", "led4", "led5", "led6", "led7", "led8", "durchR", "durchG", "durchB", "AF", "Laser0", "Laser1", "Laser2", "Laser3", "Laser4", "LaserX", "TrigOut", "SMB1", ""}
  T20 = cluster{"rel 10µs":u32, "Device":T10, "data0":i32, "data1":i32, "data2":i32, "data3":i32, "data4":i32, "data5":i32}[]
  T21 = typedef "ScanControl.ctl" = cluster{"Time [s]":dbl, "action":T5, "channel":T3, "value (/s)":dbl}[]
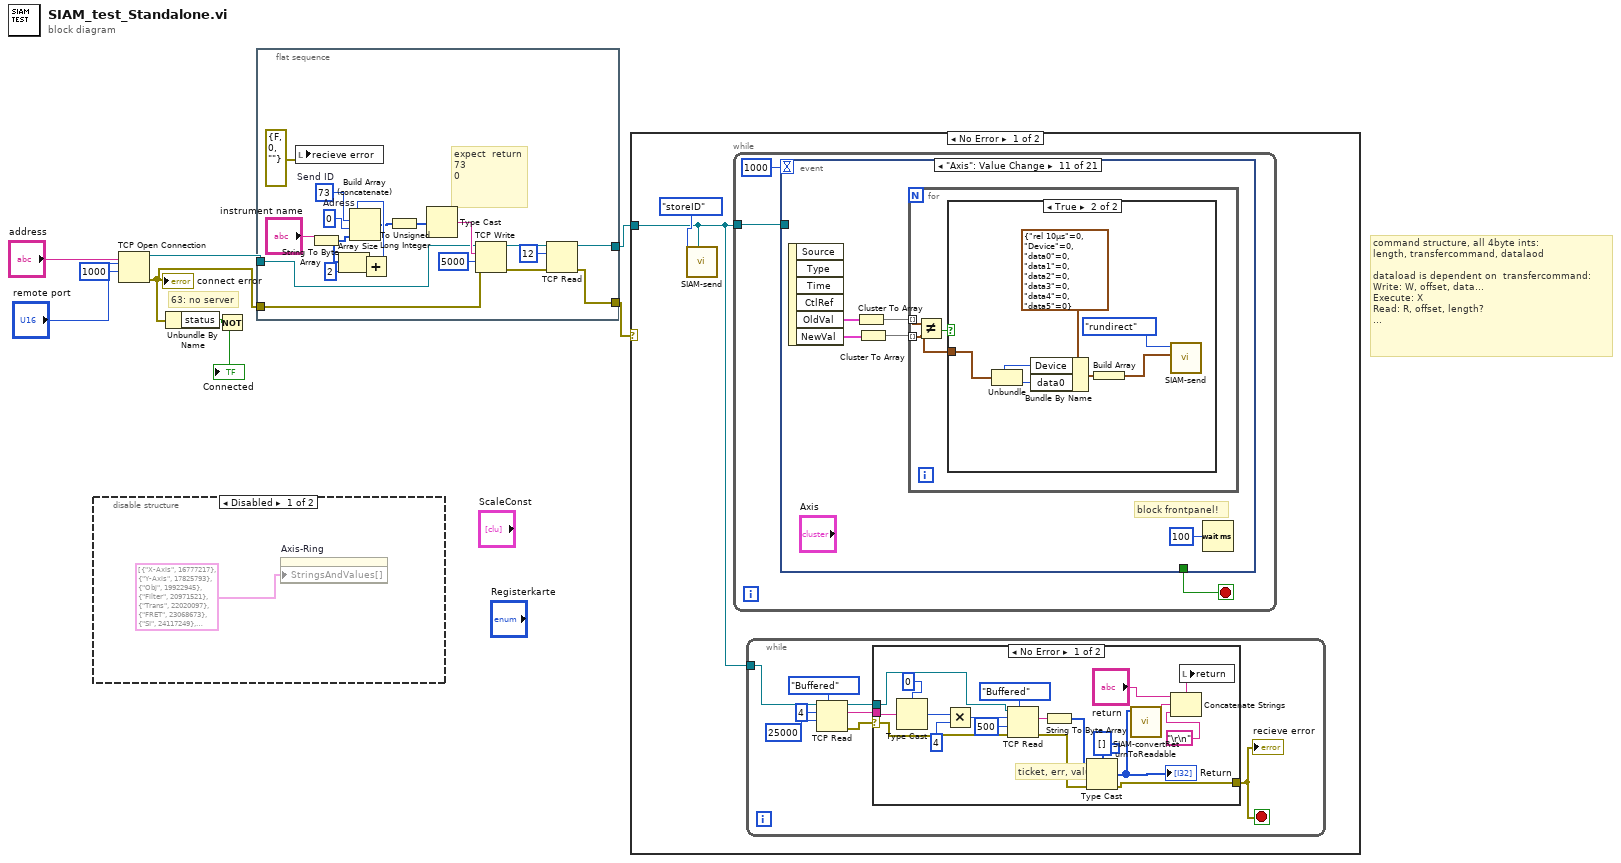
[diagram p0: block diagram]
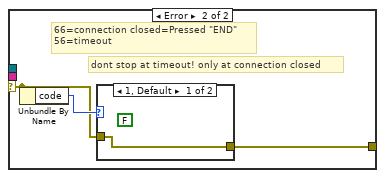
[diagram p3: hidden frame]
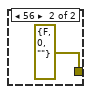
[diagram p4: hidden frame]
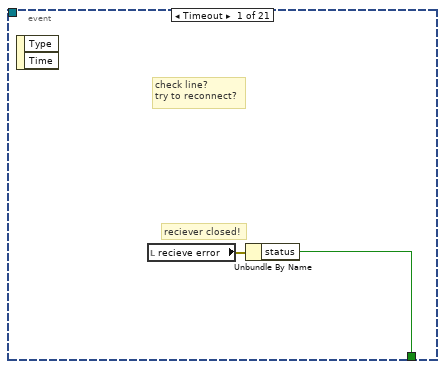
[diagram p5: hidden frame]
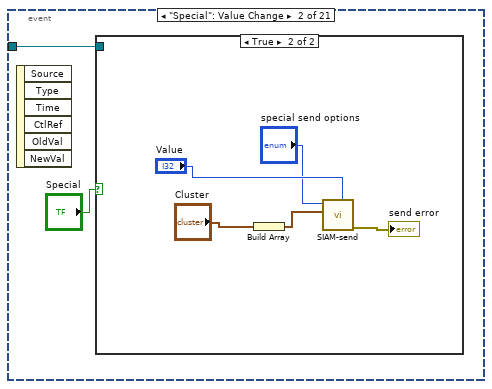
[diagram p6: hidden frame]
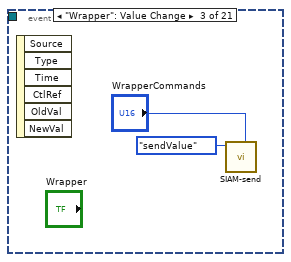
[diagram p8: hidden frame]
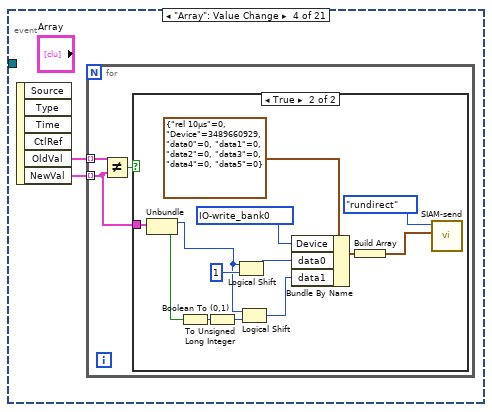
[diagram p9: hidden frame]
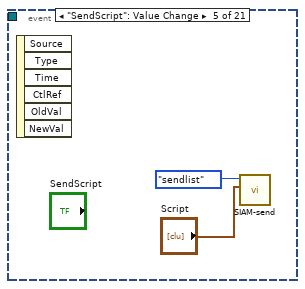
[diagram p11: hidden frame]
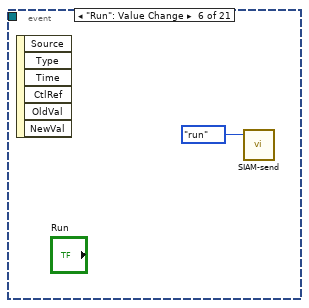
[diagram p12: hidden frame]
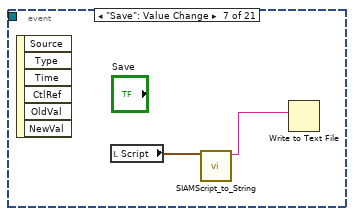
[diagram p13: hidden frame]
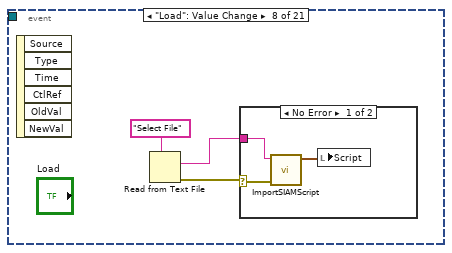
[diagram p14: hidden frame]
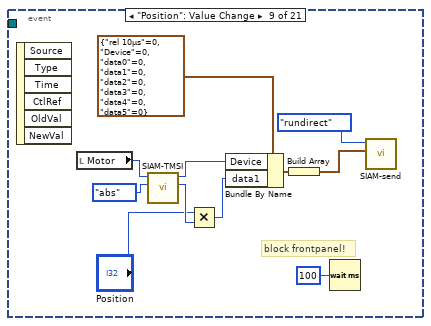
[diagram p16: hidden frame]
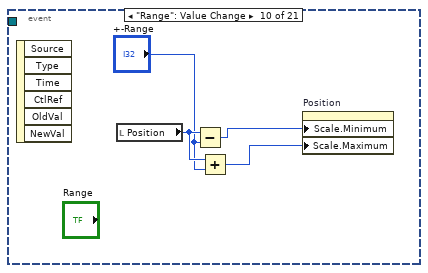
[diagram p17: hidden frame]
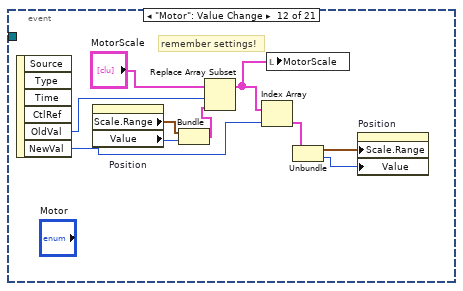
[diagram p19: hidden frame]
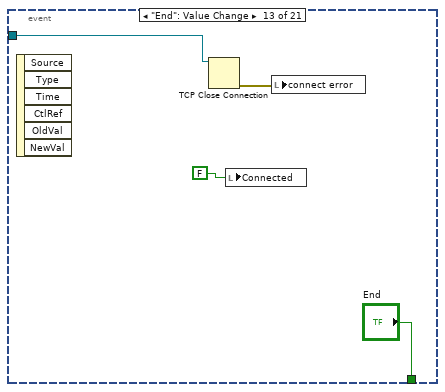
[diagram p20: hidden frame]
diagram:
  # "63: no server"
  # "command structure, all 4byte ints:\nlength, transfercommand, datalaod\n\ndataload is dependent on  transfercommand:\nWrite: W, offset, data...\nExecute: X\nRead: R, offset, length?\n..."
  n1 = disable-structure shown="Disabled" {
    frame Disabled {
      n2 = property on="Axis-Ring" class="Ring (strict)"("StringsAndValues[]"=cluster{"String":string, "command":T10}[] [{"String"="X-Axis", "command"=16777217}, {"String"="Y-Axis", "command"=17825793}, {"String"="Obj", "command"=19922945}, {"String"="Filter", "command"=20971521}, {"String"="Trans", "command"=22020097}, {"String"="FRET", "command"=23068673}, {"String"="SI", "command"=24117249}, {"String"="LED365", "command"=2684354561}, {"String"="LED385", "command"=2685403137}, {"String"="LED440", "command"=2686451713}, {"String"="LED470", "command"=2687500289}, {"String"="LED510", "command"=2688548865}, {"String"="LED540", "command"=2689597441}, {"String"="LED590", "command"=2690646017}, {"String"="LED640", "command"=2691694593}, {"String"="DurchR", "command"=2701131777}, {"String"="DurchG", "command"=2702180353}, {"String"="DurchB", "command"=2703228929}, {"String"="AF", "command"=2704277505}, {"String"="Laser0", "command"=2717908993}, {"String"="Laser1", "command"=2718957569}, {"String"="Laser2", "command"=2720006145}, {"String"="Laser3", "command"=2721054721}, {"String"="Servo0", "command"=67108865}, {"String"="Servo1", "command"=68157441}] ("Direct names")) -> ()  [unwired: 2 in, 2 out]
    }
    frame Enabled {
    }
  }
  n3 = TCP Open Connection(address="address", remote port or service name="remote port", timeout ms (60000)=1000) -> (connection ID=w3:refnum<k5>, error out=w4:errorcluster)  [unwired: 1 in, 1 out]
  "connect error" <- w4
  n4 = Unbundle By Name(w4) -> ("status"=w7:bool)
  n5 = Not(x=w7) -> (.not. x?=→"Connected":bool)
  n6 = flat-sequence {
    tunnel: w3 -> [w24]
    tunnel: w4 -> [w23]
    tunnel: [w12] -> w1
    tunnel: [w14] -> w2
    frame #0 {
      w20 = 0  # Adress
      w25 = u8 73  # Send ID
      # "expect  return\n73\n0"
      n7 = local write "recieve error"(errorcluster {"status"=FALSE, "code"=0, "source"=""} ("recieve error")) -> ()
      n8 = String To Byte Array(string="instrument name") -> (unsigned byte array=w19:u8[])
      n9 = Array Size(array=w19) -> (size(s)=w26:i32)
      n10 = Add(x=w26, y=2) -> (x+y=w17:i32)
      n11 = Build Array (concatenate)(w17, w25, w20, w19) -> (w16:i32[])
      n12 = To Unsigned Long Integer(number=w16) -> (unsigned 32bit integer=w27:u32[])
      n13 = Type Cast(x=w27) -> (*(type *) &x=w28:string)  [unwired: 1 in]
      n14 = TCP Write(connection ID=w24, data in=w28, error in (no error)=w23, 9:5000 ("timeout ms (25000)")) -> (connection ID out=w15:refnum<k5>, error out=w13:errorcluster)  [unwired: 1 out]
      n15 = TCP Read(connection ID=w15, bytes to read=12, error in (no error)=w13) -> (connection ID out=w14:refnum<k5>, error out=w12:errorcluster)  [unwired: 2 in, 1 out]
    }
  }
  n16 = case shown="No Error" w1 {
    selector: w1 -> [_ w190]
    tunnel: w2 -> [w30 w192]
    frame No Error {
      n17 = call "SIAM-send.vi"("connection ID"=w30, "command"=SIAM-send."storeID") -> ()  [unwired: 8 in, 2 out]
      n18 = while {
        tunnel: w30 -> [w64]
        stop <- w65 stop-if-true
        n19 = event shown="[10] \"Axis\": Value Change" {
          selector: _ -> [_ _ _ _ _ _ _ _ _ _ _ _ _ _ _ _ _ _ _ _ _]
          dyn-events: _ -> [_ _ _ _ _ _ _ _ _ _ _ _ _ _ _ _ _ _ _ _ _]
          timeout: 1000 -> [_ _ _ _ _ _ _ _ _ _ _ _ _ _ _ _ _ _ _ _ _]
          tunnel: [w66 _ _ _ _ _ _ _ _ _ _ _ "End" FALSE _ _ _ _ _ _ _] -> w65
          tunnel: w64 -> [_ w68 _ _ _ _ _ _ _ _ _ _ w148 _ _ _ _ _ _ _ _]
          event Timeout {
            # "reciever closed!"
            # "check line?\ntry to reconnect?"
            n20 = event-data() -> ()  [unwired: 3 out]
            n21 = local read "recieve error"() -> (w67:errorcluster)
            n22 = Unbundle By Name(w67) -> ("status"=w66:bool)
          }
          event "Special": Value Change {
            n23 = event-data() -> ()  [unwired: 7 out]
            n24 = case shown="True" "Special" {
              tunnel: w68 -> [_ _]
              frame False {
              }
              frame True {
                n25 = Build Array("Cluster") -> (w70:T11)
                n26 = call "SIAM-send.vi"("Value"="Value", "Script"=w70, "command"="special send options") -> ("error out"=→"send error":errorcluster)  [unwired: 7 in, 1 out]
              }
            }
          }
          event "Wrapper": Value Change {
            n27 = event-data() -> ()  [unwired: 7 out]
            n28 = call "SIAM-send.vi"("Value"="WrapperCommands", "command"=SIAM-send."sendValue") -> ()  [unwired: 8 in, 2 out]
          }
          event "Array": Value Change {
            n29 = event-data() -> ("OldVal"=w78:T9, "NewVal"=w77:T9)  [unwired: 5 out]
            n30 = for {
              tunnel: w78 -> [w81] mode=indexing
              tunnel: w77 -> [w79] mode=indexing
              n31 = Not Equal?(x=w81, y=w79) -> (x != y?=w80:bool)
              n32 = case shown="True" w80 {
                tunnel: w79 -> [_ w84]
                frame False {
                }
                frame True {
                  w86 = T10 3489660929 items=["read_x-Motor_status_ticket"=17305600, "init_x-Motor"=17760263, "read_x-Motor_absolute_ticket"=16781312, "move_x-Motor_absolute"=16777217, "move_x-Motor_relative"=16842753, "read_y-Motor_status_ticket"=18354176, "init_y-Motor"=18808839, "read_y-Motor_absolute_ticket"=17829888, "move_y-Motor_absolute"=17825793, "move_y-Motor_relative"=17891329, "read_z-Motor_status_ticket"=19402752, "init_z-Motor"=19857415, "stop_z-Motor"=19857423, "start_z-Motor"=19857422, "read_z-Motor_absolute_ticket"=18878464, "move_z-Motor_absolute"=18874369, "move_z-Motor_relative"=18939905, "read_Objective_status_ticket"=20451328, "init_Objective"=20905991, "read_Objective_absolute_ticket"=19927040, "move_Objective_absolute"=19922945, "move_Objective_relative"=19988481, "read_Filter_status_ticket"=21499904, "init_Filter"=21954567, "read_Filter_absolute_ticket"=20975616, "move_Filter_absolute"=20971521, "move_Filter_relative"=21037057, "read_Trans-Rad_status_ticket"=22548480, "init_Trans-Rad"=23003143, "read_Trans-Rad_absolute_ticket"=22024192, "move_Trans-Rad_absolute"=22020097, "move_Trans-Rad_relative"=22085633, "read_FRET_status_ticket"=23597056, "init_FRET"=24051719, "read_FRET_absolute_ticket"=23072768, "move_FRET_absolute"=23068673, "move_FRET_relative"=23134209, "read_SI-Rad_status_ticket"=24645632, "init_SI-Rad"=25100295, "read_SI-Rad_absolute_ticket"=24121344, "move_SI-Rad_absolute"=24117249, "move_SI-Rad_relative"=24182785, "end_no_ticket"=4027514895, "end_ticket"=4027518991, "IO-read_bank0"=3489665024, "IO-write_bank0"=3489660929, "IO-read_bank1"=3506442240, "IO-write_bank1"=3506438145, "Analog-write_DA0-0"=2684354561, "Analog-write_DA0-1"=2685403137, "Analog-write_DA0-2"=2686451713, "Analog-write_DA0-3"=2687500289, "Analog-write_DA0-4"=2688548865, "Analog-write_DA0-5"=2689597441, "Analog-write_DA0-6"=2690646017, "Analog-write_DA0-7"=2691694593, "Analog-write_DA1-0"=2701131777, "Analog-write_DA1-1"=2702180353, "Analog-write_DA1-2"=2703228929, "Analog-write_DA1-3"=2704277505, "Analog-write_DA1-4"=2705326081, "Analog-write_DA1-5"=2706374657, "Analog-write_DA1-6"=2707423233, "Analog-write_DA1-7"=2708471809, "Analog-read_AD0-0"=2818576384, "Analog-read-store_AD0-0"=2818572290, "IO-delay_bank0"=3489923073, "IO-delay_bank0_fromVar"=3489923075, "read_cam_clock"=3289124864, "store_cam_clock"=3289120770, "read_cam_phase"=3289190400, "set_cam_deadtime"=3288989697, "set_cam_10uscycles"=3289055233, "set_cam_10uscycles_fromVariable"=3289055235, "calc_cam"=3289317386, "store_cam_Var"=3289251842, "math_addToVariable"=4060086278, "readVar"=4060090368, "writeVar"=4060086273, "copyVar"=4060086276, "decrement_branchRel_if_equal"=4043374945, "decrement_branchRel_if_greaterequal"=4043375201, "decrement_branchRel_if_greaterequal_withTicket"=4043379297, "decrement_branchRel_if_smaller"=4043375457, "increment_branchRel_if_smaller"=4043375473, "set_1Galvo"=101712113, "set_x-Galvo"=102760689, "set_y-Galvo"=103809265, "set_z-Fokus"=104857841, "set_1Galvo_position-only"=101711937, "set_x-Galvo_position-only"=102760513, "set_y-Galvo_position-only"=103809089, "set_z-Fokus_position-only"=104857665, "set_x-Galvo_position-only_ticket"=102764609, "set_y-Galvo_position-only_ticket"=103813185, "set_z-Fokus_position-only_ticket"=104861761, "set_x-Galvo_relativ-only"=102760577, "set_y-Galvo_relativ-only"=103809153, "set_z-Fokus_relativ-only"=104857729, "set_x-Galvo_speed-only"=102760481, "set_y-Galvo_speed-only"=103809057, "set_z-Fokus_speed-only"=104857633, "read_1Galvo_ticket"=101716032, "read_x-Galvo_ticket"=102764608, "read_y-Galvo_ticket"=103813184, "read_z-Focus_ticket"=104861760, "x-Galvo_pos_fromVar"=102760515, "y-Galvo_pos_fromVar"=103809091, "z-Focus_pos_fromVar"=104857667, "Servo0"=67108865, "Servo1"=68157441, "Servo2"=69206017] ("Device")
                  n33 = Unbundle(w84) -> ("Digital-out"=w83:T19, "Boolean"=w82:bool)
                  n34 = Boolean To (0,1)(Boolean=w82) -> (0, 1=w89:i16)
                  n35 = To Unsigned Long Integer(number=w89) -> (unsigned 32bit integer=w85:u32)
                  n36 = Logical Shift(y=w83, x=u32 1) -> (x << y=w88:u32)
                  n37 = Logical Shift(y=w83, x=w85) -> (x << y=w87:u32)
                  n38 = Bundle By Name(cluster=T16 {"rel 10µs"=0, "Device"=3489660929, "data0"=0, "data1"=0, "data2"=0, "data3"=0, "data4"=0, "data5"=0} ("output cluster"), "Device"=w86, "data0"=w88, "data1"=w87) -> (w94:T16)
                  n39 = Build Array(w94) -> (w93:T20)
                  n40 = call "SIAM-send.vi"("Script"=w93, "command"=SIAM-send."rundirect") -> ()  [unwired: 8 in, 2 out]
                }
              }
            }
          }
          event "SendScript": Value Change {
            n41 = event-data() -> ()  [unwired: 7 out]
            n42 = call "SIAM-send.vi"("Script"="Script", "command"=SIAM-send."sendlist") -> ()  [unwired: 8 in, 2 out]
          }
          event "Run": Value Change {
            n43 = event-data() -> ()  [unwired: 7 out]
            n44 = call "SIAM-send.vi"("command"=SIAM-send."run") -> ()  [unwired: 9 in, 2 out]
          }
          event "Save": Value Change {
            n45 = event-data() -> ()  [unwired: 7 out]
            n46 = local read "Script"() -> (w99:T11)
            n47 = call "SIAMScript_to_String.vi"("Script"=w99) -> ("String"=w98:string)  [unwired: 9 in, 1 out]
            n48 = Write to Text File(text=w98) -> ()  [unwired: 3 in, 3 out]
          }
          event "Load": Value Change {
            n49 = event-data() -> ()  [unwired: 7 out]
            n50 = Read from Text File(prompt (Open existing file)="Select File") -> (text=w101:string, error out=w100:errorcluster)  [unwired: 3 in, 2 out]
            n51 = case shown="No Error" w100 {
              selector: w100 -> [w103 _]
              tunnel: w101 -> [w104 _]
              frame No Error {
                n52 = call "ImportSIAMScript.vi"("error in (no error)"=w103, "String"=w104) -> ("Script"=w105:T11)  [unwired: 8 in, 1 out]
                n53 = local write "Script"(w105) -> ()
              }
              frame Error {
              }
            }
          }
          event "Position": Value Change {
            # "block frontpanel!"
            n54 = event-data() -> ()  [unwired: 7 out]
            n55 = local read "Motor"() -> (w106:T7)
            n56 = call "SIAM-TMSI.vi"("Type"=enum8{"acc", "vel", "abs", "offset"}."abs", "Motor"=w106) -> ("Resolution-Factor"=w112:i32, "command"=w108:T10)  [unwired: 6 in, 2 out]
            n57 = Multiply(x="Position", y=w112) -> (x*y=w110:i32)
            n58 = Bundle By Name(cluster=T16 {"rel 10µs"=0, "Device"=0, "data0"=0, "data1"=0, "data2"=0, "data3"=0, "data4"=0, "data5"=0} ("output cluster"), "Device"=w108, "data1"=w110) -> (w116:T16)
            n59 = Build Array(w116) -> (w115:T20)
            n60 = Wait (ms)(milliseconds to wait=u32 100) -> ()  [unwired: 1 out]
            n61 = call "SIAM-send.vi"("Script"=w115, "command"=SIAM-send."rundirect") -> ()  [unwired: 8 in, 2 out]
          }
          event "Range": Value Change {
            n62 = event-data() -> ()  [unwired: 7 out]
            n63 = local read "Position"() -> (w120:i32)
            n64 = Subtract(x=w120, y="+-Range") -> (x-y=w118:i32)
            n65 = Add(x=w120, y="+-Range") -> (x+y=w117:i32)
            n66 = property on="Position" class="Slide (strict)"("Scale.Minimum"=w118, "Scale.Maximum"=w117) -> ()  [unwired: 2 in, 2 out]
          }
          event "Axis": Value Change {
            # "block frontpanel!"
            n67 = event-data() -> ("OldVal"=w124:T8, "NewVal"=w123:T8)  [unwired: 5 out]
            n68 = Cluster To Array(cluster=w124) -> (array=w121:cluster{"Axis-Ring":u32, "Position":i32}[])
            n69 = Cluster To Array(cluster=w123) -> (array=w122:cluster{"Axis-Ring":u32, "Position":i32}[])
            n70 = for {
              tunnel: w121 -> [w128] mode=indexing
              tunnel: w122 -> [w127] mode=indexing
              n71 = Not Equal?(x=w128, y=w127) -> (x != y?=w126:bool)
              n72 = case shown="True" w126 {
                tunnel: w127 -> [_ w131]
                frame False {
                }
                frame True {
                  n73 = Unbundle(w131) -> ("Axis-Ring"=w130:u32, "Position"=w129:i32)
                  n74 = Bundle By Name(cluster=T16 {"rel 10µs"=0, "Device"=0, "data0"=0, "data1"=0, "data2"=0, "data3"=0, "data4"=0, "data5"=0} ("output cluster"), "Device"=w130, "data0"=w129) -> (w135:T16)
                  n75 = Build Array(w135) -> (w134:T20)
                  n76 = call "SIAM-send.vi"("Script"=w134, "command"=SIAM-send."rundirect") -> ()  [unwired: 8 in, 2 out]
                }
              }
            }
            n77 = Wait (ms)(milliseconds to wait=u32 100) -> ()  [unwired: 1 out]
          }
          event "Motor": Value Change {
            # "remember settings!"
            n78 = event-data() -> ("OldVal"=w145:T7, "NewVal"=w144:T7)  [unwired: 5 out]
            n79 = property on="Position" class="Slide (strict)"() -> ("Scale.Range"=w141:T14, "Value"=w142:i32)  [unwired: 2 in, 2 out]
            n80 = Bundle("Scale.Range"=w141, "Value"=w142) -> (w140:cluster{"Scale.Range":T14, "Value":i32})  [unwired: 1 in]
            n81 = Replace Array Subset(array="MotorScale", new element=w140, index=w145) -> (w138:cluster{"Scale.Range":T14, "Value":i32}[])
            n82 = Index Array(array=w138, index=w144) -> (element=w143:cluster{"Scale.Range":T14, "Value":i32})
            n83 = local write "MotorScale"(w138) -> ()
            n84 = Unbundle(w143) -> ("Scale.Range"=w137:T14, "Value"=w136:i32)
            n85 = property on="Position" class="Slide (strict)"("Scale.Range"=w137, "Value"=w136) -> ()  [unwired: 2 in, 2 out]
          }
          event "End": Value Change {
            n86 = event-data() -> ()  [unwired: 7 out]
            n87 = TCP Close Connection(connection ID=w148) -> (error out=w147:errorcluster)  [unwired: 1 in, 2 out]
            n88 = local write "Connected"(FALSE ("Connected")) -> ()
            n89 = local write "connect error"(w147) -> ()
          }
          event "Create": Value Change {
            n90 = event-data() -> ()  [unwired: 7 out]
            n91 = case shown="True" "Create" {
              frame False {
              }
              frame True {
                n92 = call "Galvo-TestScripts.vi"("Type"=T17."triangle", "channel"="channel", "Amplitude"="Amplitude \n(count pk-pk)", "Frequency[Hz]"="Frequency [Hz]", "Offset"="Offset [count]", "Duration [s]"="duration [s]") -> ("ScanSteuerung"=w154:T21)  [unwired: 1 in, 1 out]
                n93 = local read "TMSI-device-scales"() -> (w152:T4)
                n94 = for {
                  shift-right: [w167] -> w153
                  shift-left: w154 -> [w168]
                  tunnel: w152 -> [w166] mode=indexing
                  n95 = Unbundle(w166) -> ("channel"=w165:T3, "m/bit"=w164:dbl)  [unwired: 3 out]
                  n96 = Reciprocal(x=w164) -> (1/x=w163:dbl)
                  n97 = call "ScanSteuerung_WertSkalierung.vi"("ScanSteuerung"=w168, "Channel"=w165, "/Skalierung (m/bit)"=w163) -> ("ScanSteuerungOut"=w167:T21)  [unwired: 1 in]
                }
                n98 = call "ScanSteuerung_AndereZeitbasis.vi"("ScanSteuerung"=w153, "Neues Zeitraster"=100000.0) -> ("ScanSteuerungOut"=w155:T21)
                n99 = local write "ScanSteuerung"(w155) -> ()
              }
            }
          }
          event "ClearScan": Value Change {
            n100 = event-data() -> ()  [unwired: 7 out]
            n101 = local write "ScanSteuerung"(T18 [] ("ScanSteuerung")) -> ()
          }
          event "Update length": Value Change {
            n102 = event-data() -> ()  [unwired: 7 out]
            n103 = local read "ScanSteuerung"() -> (w171:T6)
            n104 = Array Size(array=w171) -> (size(s)=→"Elements":i32)
          }
          event "Unroll-loops": Value Change {
            n105 = event-data() -> ()  [unwired: 7 out]
            n106 = local read "ScanSteuerung"() -> (w173:T6)
            n107 = call "ScanSteuerung_RemoveLoops.vi"("ScanSteuerung"=w173) -> ("ScanSteuerungOut"=w172:T21)  [unwired: 2 out]
            n108 = local write "ScanSteuerung"(w172) -> ()
          }
          event "Clear": Value Change {
            n109 = event-data() -> ()  [unwired: 7 out]
            n110 = case shown="True" "Clear" {
              frame False {
              }
              frame True {
                n111 = local write "return"("") -> ()
              }
            }
          }
          event "ClearScript": Value Change {
            n112 = event-data() -> ()  [unwired: 7 out]
            n113 = local write "Script"(T11 [] ("Script")) -> ()
          }
          event "ConvertScan": Value Change {
            n114 = event-data() -> ()  [unwired: 7 out]
            n115 = call "ScanSteuerung_AndereZeitbasis.vi"("ScanSteuerung"="ScanSteuerung", "Neues Zeitraster"="Cycletime [s]") -> ("ScanSteuerungOut"=w180:T21)
            n116 = for {
              shift-right: [w186] -> w178
              shift-left: w180 -> [w187]
              tunnel: "TMSI-device-scales" -> [w185] mode=indexing
              n117 = Unbundle(w185) -> ("channel"=w184:T3, "m/bit"=w183:dbl)  [unwired: 3 out]
              n118 = call "ScanSteuerung_WertSkalierung.vi"("ScanSteuerung"=w187, "Channel"=w184, "/Skalierung (m/bit)"=w183) -> ("ScanSteuerungOut"=w186:T21)  [unwired: 1 in]
            }
            n119 = call "ScanControl_to_SIAM.vi"("ScanSteuerung"=w178) -> ("Script"=w181:T11)  [unwired: 2 in, 8 out]
            n120 = local write "Script"(w181) -> ()
          }
          event "Convert String": Value Change {
            n121 = event-data() -> ()  [unwired: 7 out]
            n122 = call "String2ScanSteuerung.vi"("String"="Colibri-Scan-String") -> ("ScanSteuerung"=w188:T21)
            n123 = local write "ScanSteuerung"(w188) -> ()
          }
        }
      }
      n124 = while {
        tunnel: w30 -> [w39]
        stop <- w32 stop-if-true
        n125 = TCP Read(connection ID=w39, bytes to read=4, 7:T15."Buffered" ("mode (standard)"), 9:25000 ("timeout ms (25000)")) -> (connection ID out=w35:refnum<k5>, data out=w36:string, error out=w33:errorcluster)  [unwired: 1 in]
        n126 = case shown="No Error" w33 {
          selector: w33 -> [w53 w58]
          tunnel: w36 -> [w57 _]
          tunnel: w35 -> [w54 _]
          tunnel: [w43 w59] -> w32
          frame No Error {
            # "ticket, err, value"
            n127 = Type Cast(type=u32 0, x=w57) -> (*(type *) &x=w46:u32)
            n128 = Multiply(x=w46, y=u32 4) -> (x*y=w44:u32)
            n129 = TCP Read(connection ID=w54, bytes to read=w44, error in (no error)=w53, 7:T15."Buffered" ("mode (standard)"), 9:500 ("timeout ms (25000)")) -> (data out=w51:string, error out=w43:errorcluster)  [unwired: 1 out]
            n130 = String To Byte Array(string=w51) -> (unsigned byte array=w47:u8[])
            n131 = Type Cast(type=i32[] [], x=w47) -> (*(type *) &x=w40:i32[])
            "Return" <- w40
            n132 = call "SIAM-convertReturnToReadable.vi"("Return"=w40) -> ("Readable"=w48:string)  [unwired: 1 in, 9 out]
            n133 = Concatenate Strings("return", w48, "\r\n") -> (w50:string)
            n134 = local write "return"(w50) -> ()
          }
          frame Error {
            # "dont stop at timeout! only at connection closed"
            # "66=connection closed=Pressed \"END\"\n56=timeout"
            n135 = Unbundle By Name(w58) -> ("code"=w60:i32)
            n136 = case shown="1, Default" w60 {
              tunnel: [w61 errorcluster {"status"=FALSE, "code"=0, "source"=""} ("error out")] -> w59
              tunnel: w58 -> [w61 _]
              frame 1, Default {
                (unwired) FALSE ("Connected")
              }
              frame 56 {
              }
            }
          }
        }
        "recieve error" <- w32
      }
    }
    frame Error {
      n137 = TCP Close Connection(connection ID=w192, error in (no error)=w190) -> (error out=w191:errorcluster)  [unwired: 1 in, 1 out]
      n138 = local write "connect error"(w191) -> ()
    }
  }
